vi "LOGIC.vi"(8 "error out":errorcluster, 9 "Invert":bool, 10 "Logic Output":u16(ring)=1 items=["Not Scan / Not Reading"=1, "Shutter Open"=2, "Not Ready/Busy"=3, "Always Low"=4, "Always High"=8], 11 "Camera Handle":u32) -> (0 "error out 2":errorcluster, 1 "String":string, 2 "INI Flag":bool, 3 "Camera Handle":u32)   [LabVIEW 2015]
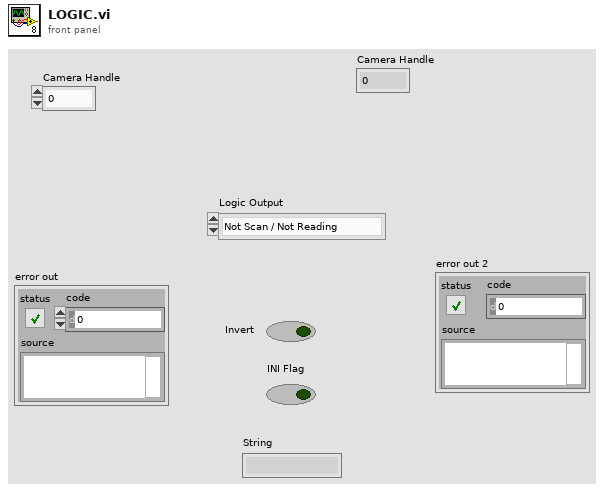
[diagram p1: front panel]
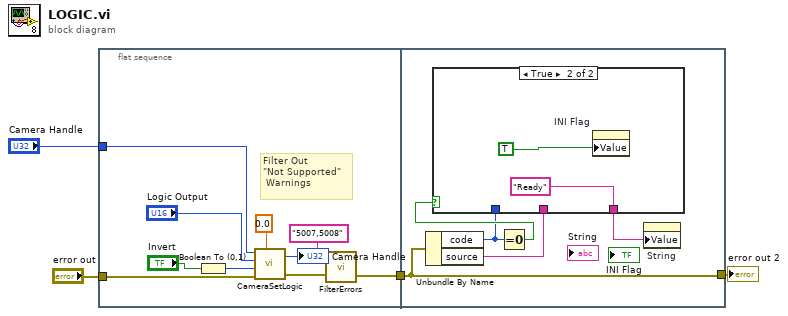
[diagram p0: block diagram]
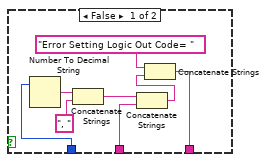
[diagram p2: hidden frame]
diagram:
  n1 = flat-sequence {
    tunnel: [w9] -> w4
    tunnel: "error out" -> [w12]
    tunnel: "Camera Handle" -> [w8]
    tunnel: w4 -> [w19]
    tunnel: [w19] -> w1
    frame #0 {
      # "Filter Out\n\"Not Supported\"\n Warnings"
      n2 = Boolean To (0,1)(Boolean="Invert") -> (0, 1=w14:i16)
      n3 = call <userlib>:"CameraSetLogic.vi"("Reserved"=0.0, "error in (no error)"=w12, "Invert Logic"=w14, "Logic Output"="Logic Output", "Camera Handle"=w8) -> ("error out"=w10:errorcluster, "Camera Handle"=→"Camera Handle":u32)  [unwired: 1 in]
      n4 = call "FilterErrors.vi"("error in (no error)"=w10, "Error Numbers To Filter"="5007,5008") -> ("error out"=w9:errorcluster)
    }
    frame #1 {
      n5 = Unbundle By Name(w19) -> ("code"=w16:i32, "source"=w17:string)
      n6 = Equal To 0?(x=w16) -> (x = 0?=w18:bool)
      n7 = case shown="True" w18 {
        tunnel: [w20 "Ready"] -> w15
        tunnel: w17 -> [w21 _]
        tunnel: w16 -> [w26 _]
        frame False {
          n8 = Number To Decimal String(number=w26) -> (decimal integer string=w25:string)  [unwired: 1 in]
          n9 = Concatenate Strings(w25, ", ") -> (w22:string)
          n10 = Concatenate Strings(w22, w21) -> (w23:string)
          n11 = Concatenate Strings("Error Setting Logic Out Code= ", w23) -> (w20:string)
        }
        frame True {
          n12 = property on="INI Flag" class="Bool (strict)"("Value"=TRUE) -> ()  [unwired: 2 in, 2 out]
        }
      }
      n13 = property on="String" class="Str"("Value"=w15) -> ()  [unwired: 2 in, 2 out]
    }
  }
  "error out 2" <- w1
